vi "Memory.Array.Subset Reference.vi"(7 "length (-1: rest)":i64=-1 format="%d bytes", 8 "error in (no error)":errorcluster, 9 "index (0)":u64, 11 "Array in":refnum<class "Memory.Array.lvclass">) -> (0 "error out":errorcluster, 2 "subset Array":refnum<class "Memory.Array.lvclass">, 3 "Array out":refnum<class "Memory.Array.lvclass">)   [LabVIEW 2016, in "LabVIEW Memory Manager.lvlib" / "Memory.Array.lvclass"]
uses:
  Memory.Array.lvclass
  Pointer/Memory.Pointer.lvclass
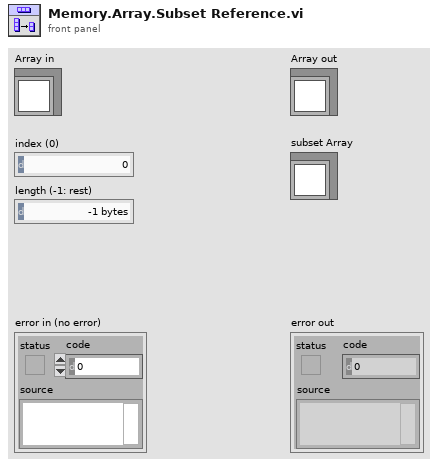
[diagram p1: front panel]
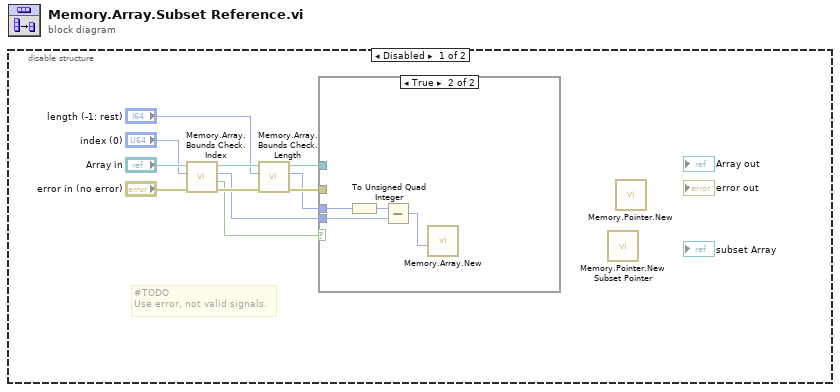
[diagram p0: block diagram]
diagram:
  n1 = disable-structure shown="Disabled" {
    frame Disabled {
      # "#TODO\nUse error, not valid signals."
      n2 = call "Memory.Array.Bounds Check.Index.vi"("error in (no error)"="error in (no error)", "index"="index (0)", "Array in"="Array in") -> ("error out"=w8:errorcluster, "index valid"=w3:bool, "index out"=w2:u64, "Array out"=w9:refnum<class "Memory.Array.lvclass">)  [unwired: 5 in]
      n3 = call "Memory.Array.Bounds Check.Length.vi"("error in (no error)"=w8, "length"="length (-1: rest)", "Array in"=w9) -> ("error out"=w5:errorcluster, "length out"=w1:i64, "Array out"=w4:refnum<class "Memory.Array.lvclass">)  [unwired: 5 in, 1 out]
      n4 = case shown="True" w3 {
        tunnel: w1 -> [_ w14]
        tunnel: w2 -> [_ w12]
        tunnel: w5 -> [_ _]
        tunnel: w4 -> [_ _]
        frame False {
        }
        frame True {
          n5 = To Unsigned Quad Integer(1:w14) -> (0:w13:u64)
          n6 = Subtract(x=w13, y=w12) -> (x-y=w15:u64)
          n7 = call "Memory.Array.New.vi"("number of elements"=w15) -> ()  [unwired: 9 in, 2 out]
        }
      }
      n8 = call "Memory.Pointer.New Subset Pointer.vi"() -> ()  [unwired: 9 in, 3 out]
      n9 = call "Memory.Pointer.New.vi"() -> ()  [unwired: 9 in, 3 out]
    }
    frame Enabled {
    }
  }
